vi "Main_Robot_Control2_j.vi"() -> ()   [LabVIEW 2014]
uses:
  <vilib>/Platform/TimedLoop/XDataNode/timing_clust.ctl
  <vilib>/Platform/TimedLoop/XDataNode/nitl_modes.ctl
  <vilib>/Platform/TimedLoop/XDataNode/wakeup.ctl
  <vilib>/Platform/TimedLoop/XDataNode/XDataNode.xnode
  <vilib>/Platform/TimedLoop/XDataNode/XDNodeRunTimeDep.lvlib
panel:
  in  "Subpanel Stop":bool
  out "Previous Iteration Finished Late?  2":bool
  out "Subpanel Running":bool
  out "Pot_D":dynamicdata(graph)
  out "IR_V":dynamicdata(graph)
  out "IR_D":dynamicdata(graph)
  out "Numeric":dbl
  out "Numeric 2":dbl
  out "Pot_V":dynamicdata(graph)
  out "stop 3":bool
  in  "stop 2":bool
  out "Boolean":bool
  in  "motor direction":bool
  in  "Set Start Posiotn of Head in Steps":dbl format="%#_13g"
  in  "Tab Control":T1(tab)
  out "Center IR":dbl(slide) scale=0.0..10.0
  out "Pot":dbl(slide) scale=0.0..10.0
  out "Gauge":dbl(knob) scale=0.0..10.0
  in  "Motor Direction":bool
  in  "Potentiometer":dbl(slide) scale=0.0..5.0
  out "Previous Iteration Finished Late?":bool
  # "E-STOP"
  # "See the block diagram for modification instructions."
  # "CCW"
  # "CCW"
  # "CW"
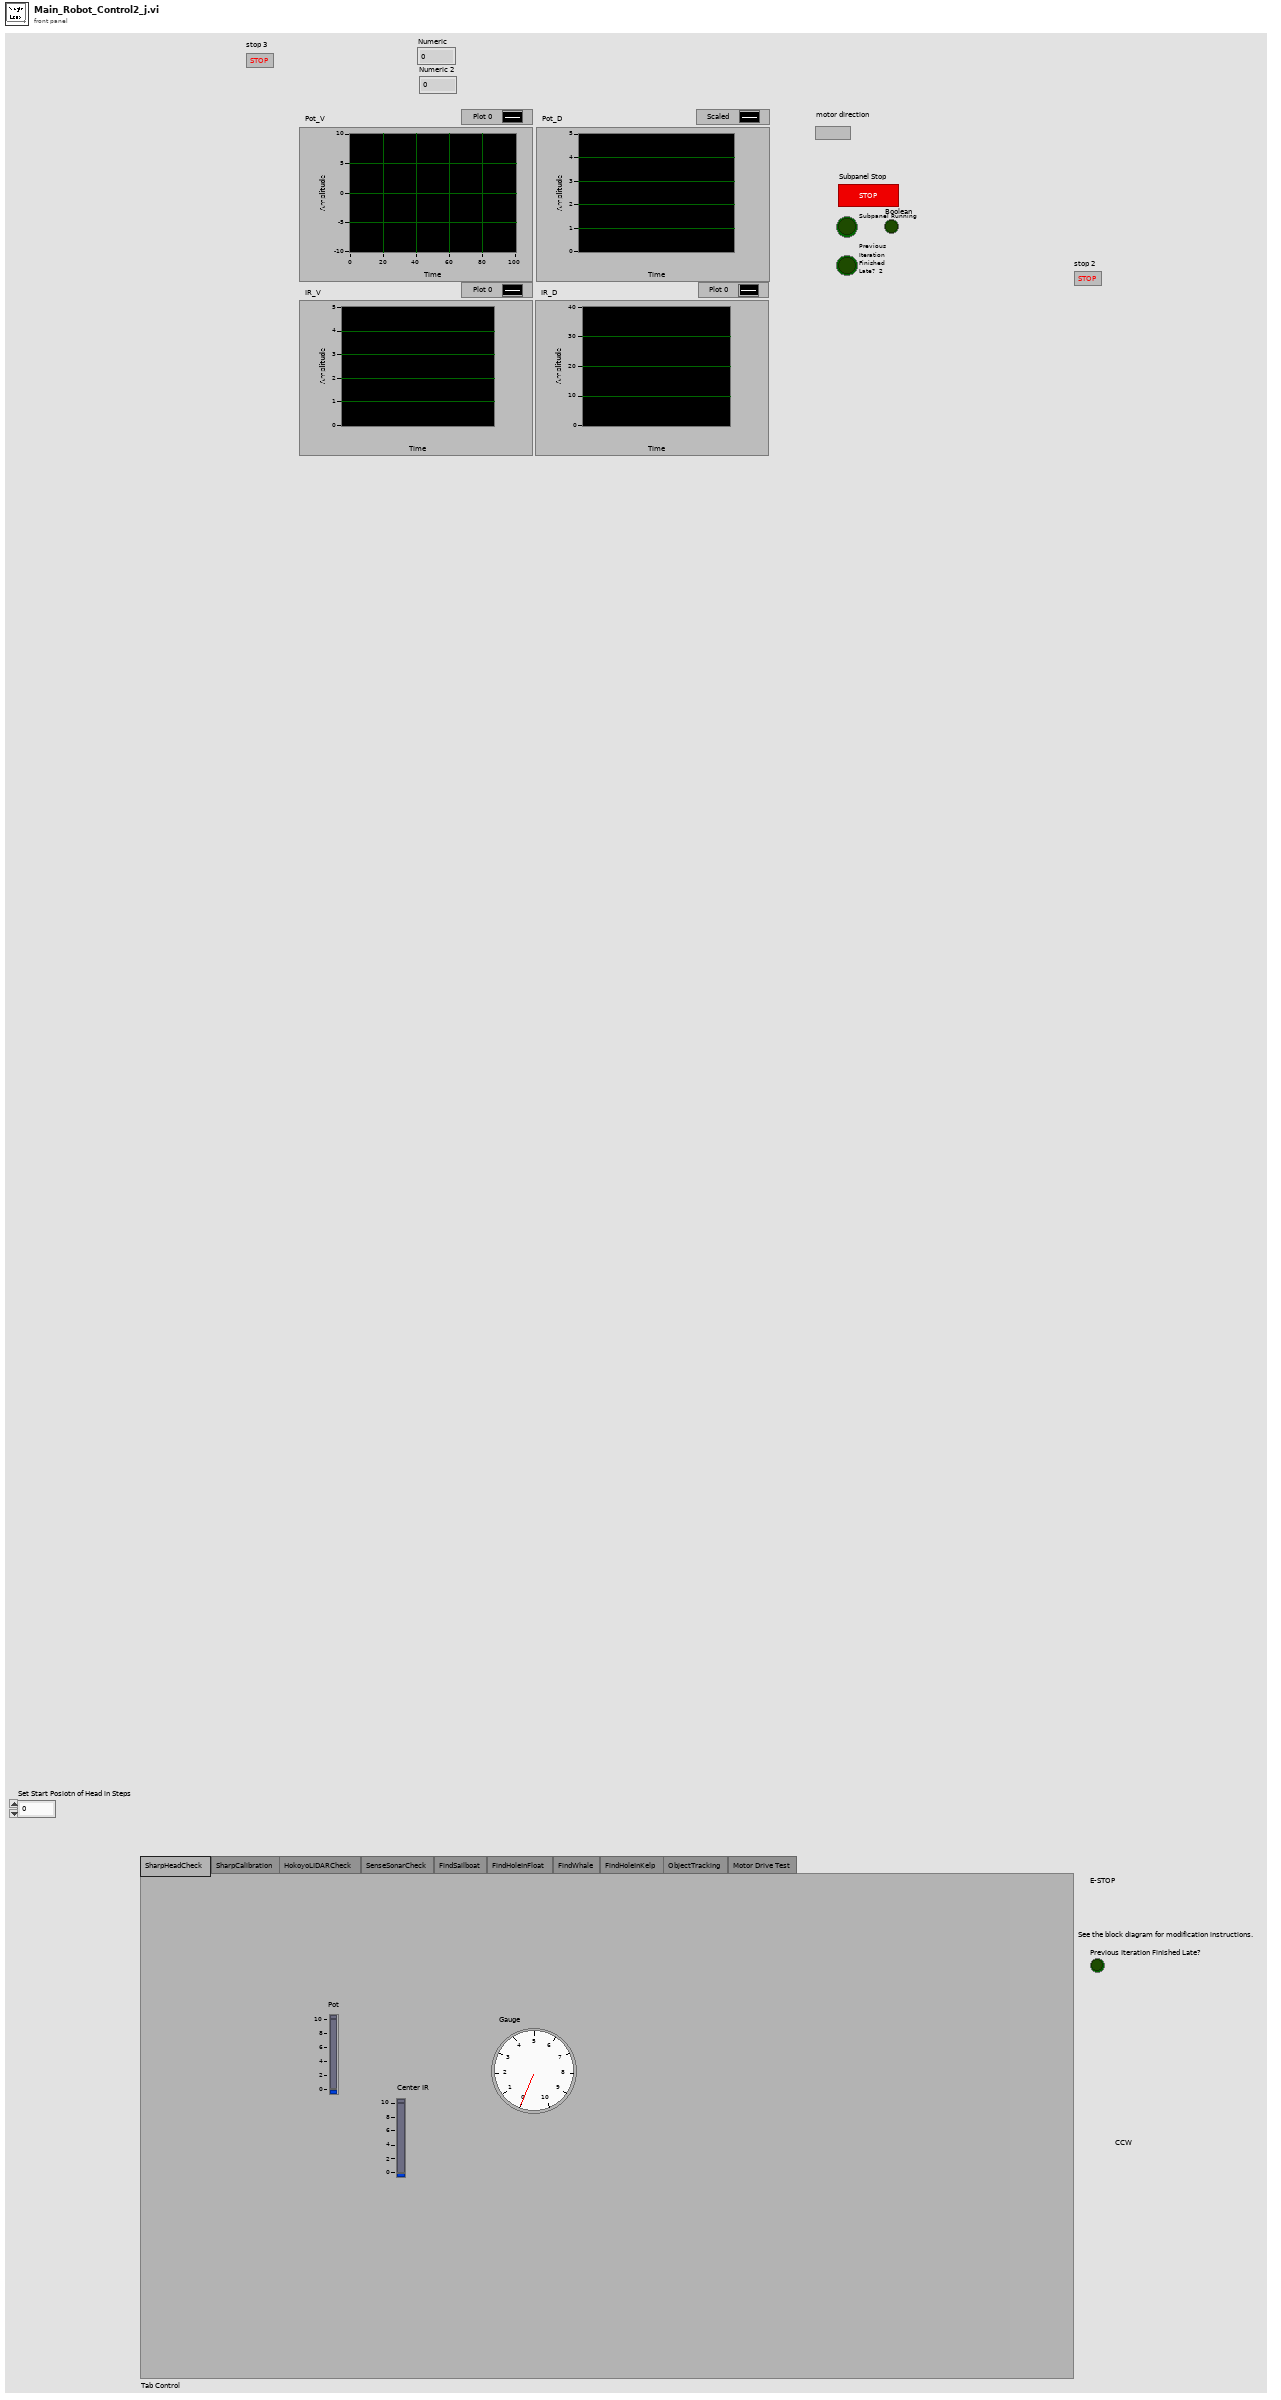
[diagram p1: front panel]
types:
  T1 = enum32{"SharpHeadCheck", "SharpCalibration", "HokoyoLIDARCheck", "SenseSonarCheck", "FindSailboat", "FindHoleInFloat", "FindWhale", "FindHoleInKelp", "ObjectTracking", "Motor Drive Test"}
  T2 = typedef "XDNodeRunTimeDep.lvlib/timing_clust.ctl" = cluster{"Expected End [f-1]":u64, "Actual End [f-1]":u64, "Finished Late? [f-1]":bool, "Expected End [i-1]":u64, "Actual End [i-1]":u64, "Finished Late? [i-1]":bool, "Expected Start [i]":u64, "Actual Start [i]":u64, "Expected Start [f]":u64, "Actual Start [f]":u64, "Source Name":string, "Structure Name":string, "Period":i64, "Deadline":i64, "Offset":i64, "Start":i64, "Priority":i32, "Timeout":i32, "Mode":T3, "Wakeup Reason":T4, "Error":errorcluster, "Source Type":string, "Secondary Source Type":string, "Global End Time":u64, "Global Start Time":u64, "Frame Duration":u64, "Iteration Duration":u64, "Assigned CPU":i32, "I/O Scan Engine Mode":u32}
  T3 = typedef "XDNodeRunTimeDep.lvlib/nitl_modes.ctl" = enum32{"No Change", "Process missed periods, maintain original phase", "Discard missed periods, maintain original phase", "Process missed periods, ignore original phase", "Discard missed periods, ignore original phase"}
  T4 = typedef "XDNodeRunTimeDep.lvlib/wakeup.ctl" = enum32{"Normal", "Aborted", "Asynchronous wakeup", "Timing source error", "Timed loop error", "Timeout"}
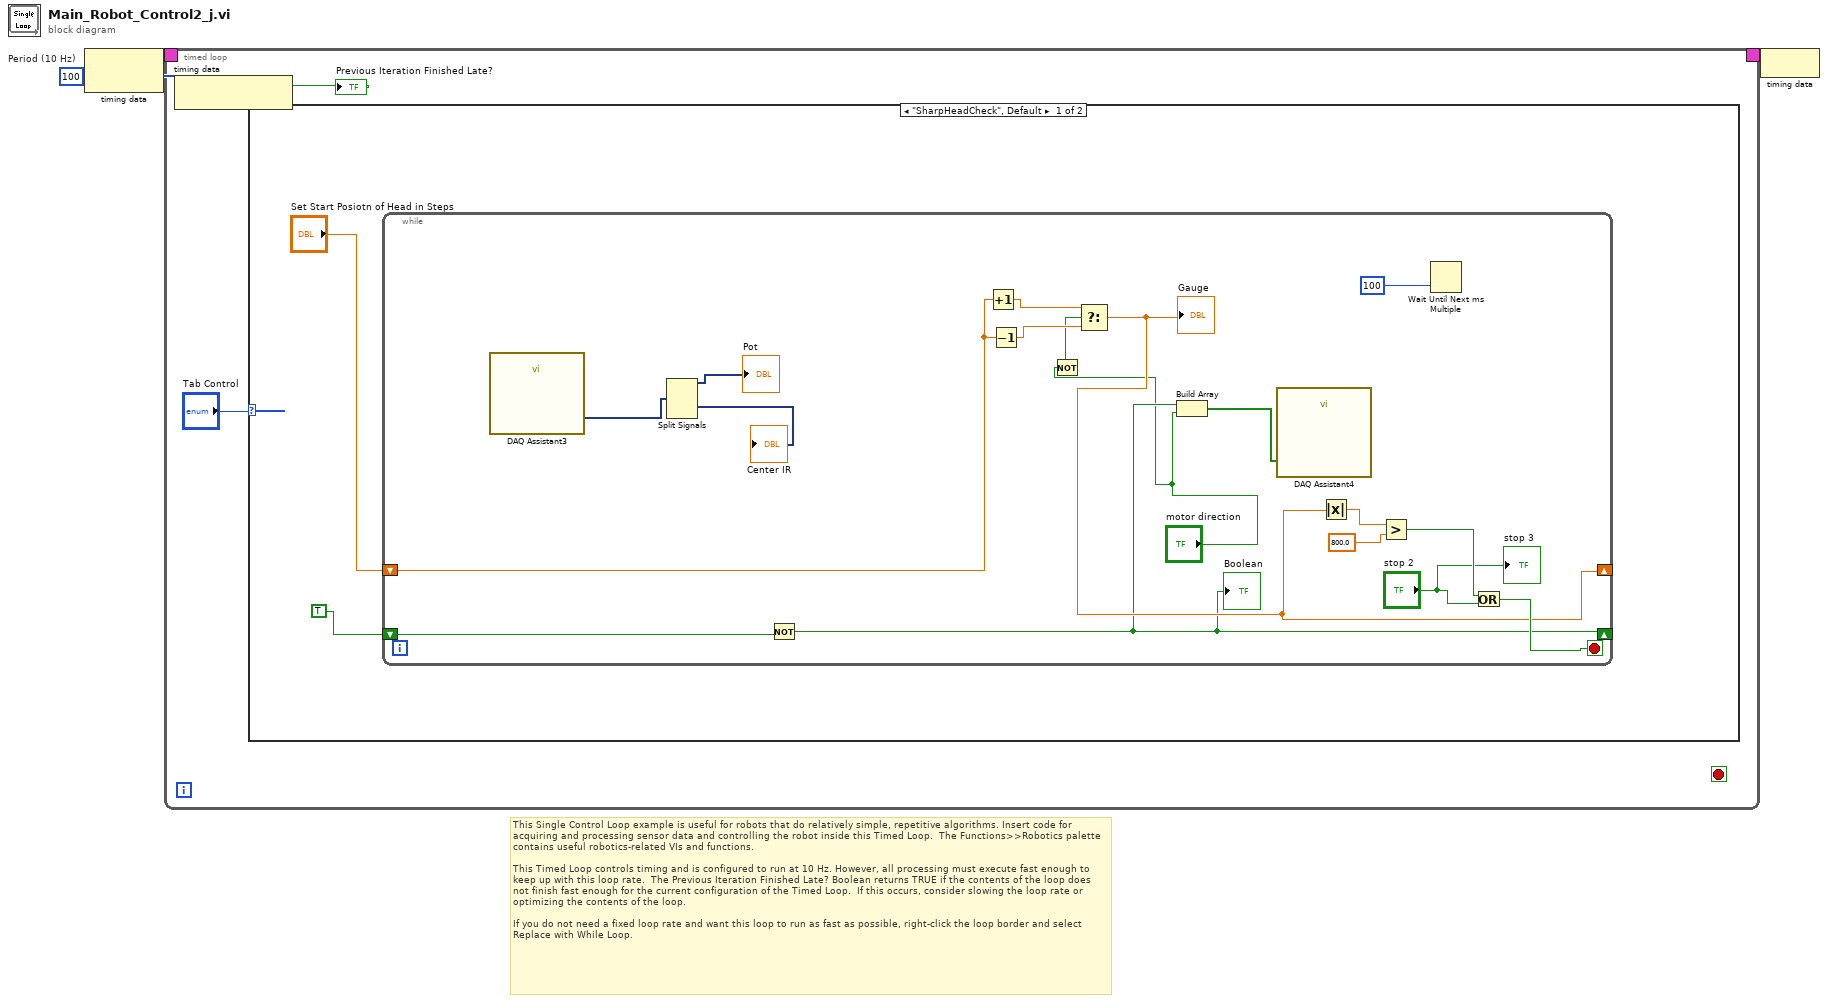
[diagram p0: block diagram]
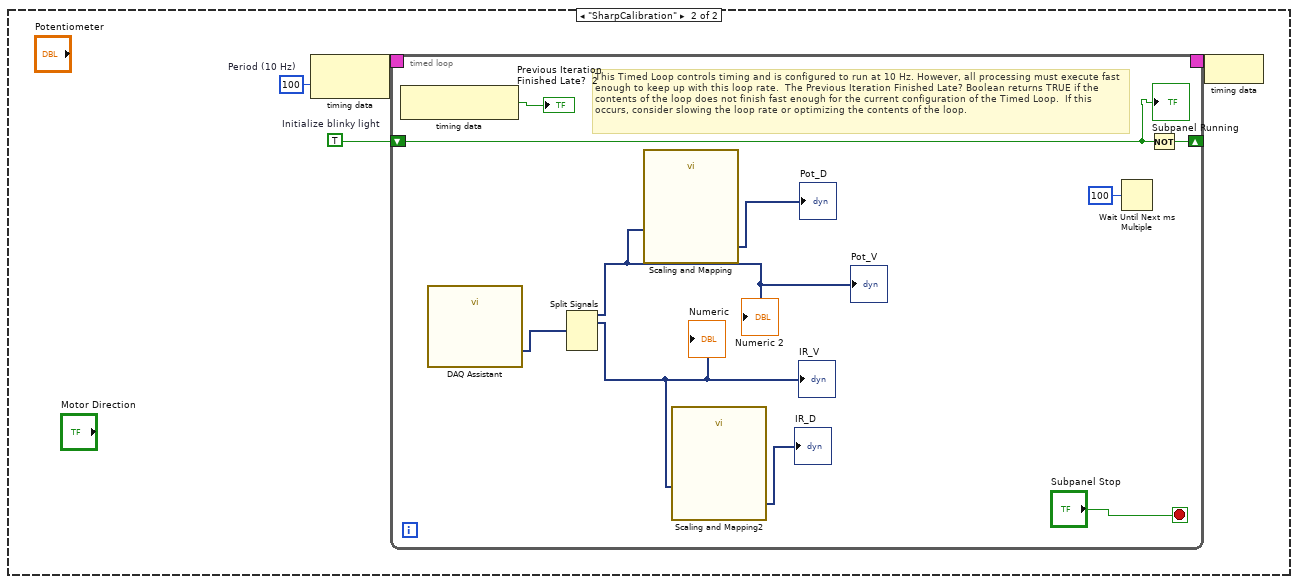
[diagram p2: hidden frame]
diagram:
  w1 = i64 100  # Period (10 Hz)
  # "This Single Control Loop example is useful for robots that do relatively simple, repetitive algorithms. Insert code for acquiring and processing sensor data and controlling the robot inside this Timed Loop.  The Functions>>Robotics palette contains useful robotics-related VIs and functions.\n\nThis Timed Loop controls timing and is configured to run at 10 Hz. However, all processing must execute fast enough to keep up with this loop rate.  The Previous Iteration Finished Late? Boolean returns TRUE if the contents of the loop does not finish fast enough for the current configuration of the Timed Loop.  If this occurs, consider slowing the loop rate or optimizing the contents of the loop.\n\nIf you do not need a fixed loop rate and want this loop to run as fast as possible, right-click the loop border and select Replace with While Loop."
  n1 = node-c288(w1) -> (w3:T2)
  n2 = timed-loop {
    timing: w3 -> [_]
    timing-out: [_] -> w2
    stop <- _ stop-if-true
    n3 = node-c288() -> (→"Previous Iteration Finished Late?":bool)  [unwired: 1 in]
    n4 = case shown="\"SharpHeadCheck\", Default" "Tab Control" {
      frame "SharpHeadCheck", Default {
        n5 = while {
          shift-right: [w13] -> _
          shift-left: TRUE -> [w18]
          shift-right: [w14] -> _
          shift-left: "Set Start Posiotn of Head in Steps" -> [w25]
          stop <- w22 stop-if-true
          n6 = call "DAQ Assistant3"() -> ("data"=w16:dynamicdata)  [unwired: 17 in, 2 out]
          n7 = Split Signals(w16) -> (→"Pot":dynamicdata, →"Center IR":dynamicdata)  [unwired: 5 in, 3 out]
          n8 = Not(x=w18) -> (.not. x?=w13:bool)
          "Boolean" <- w13
          n9 = Increment(x=w25) -> (x+1=w23:dbl)
          n10 = Decrement(x=w25) -> (x-1=w24:dbl)
          n11 = Not(x="motor direction") -> (.not. x?=w10:bool)
          n12 = Select(t=w23, s=w10, f=w24) -> (s? t:f=w14:dbl)
          "Gauge" <- w14
          n13 = Build Array(w13, "motor direction") -> (w15:bool[])
          n14 = call "DAQ Assistant4"("data"=w15) -> ()  [unwired: 17 in, 2 out]
          n15 = Absolute Value(x=w14) -> (abs(x)=w19:dbl)
          n16 = Greater?(x=w19, y=800.0) -> (0:w21:bool)
          n17 = Wait Until Next ms Multiple(millisecond multiple=u32 100 ("millisecond timer value")) -> ()  [unwired: 1 out]
          n18 = Or(x=w21, y="stop 2") -> (x .or. y?=w22:bool)
          "stop 3" <- "stop 2"
        }
      }
      frame "SharpCalibration" {
        w26 = TRUE  # Initialize blinky light
        w27 = i64 100  # Period (10 Hz)
        n19 = node-c288(w27) -> (w29:T2)
        n20 = timed-loop {
          timing: w29 -> [_]
          timing-out: [_] -> w28
          shift-right: [w39] -> _
          shift-left: w26 -> [w36]
          stop <- "Subpanel Stop" stop-if-true
          # "This Timed Loop controls timing and is configured to run at 10 Hz. However, all processing must execute fast enough to keep up with this loop rate.  The Previous Iteration Finished Late? Boolean returns TRUE if the contents of the loop does not finish fast enough for the current configuration of the Timed Loop.  If this occurs, consider slowing the loop rate or optimizing the contents of the loop."
          n21 = node-c288() -> (→"Previous Iteration Finished Late?  2":bool)  [unwired: 1 in]
          n22 = call "DAQ Assistant"() -> ("data"=w32:dynamicdata)  [unwired: 17 in, 2 out]
          n23 = Split Signals(w32) -> (w30:dynamicdata, w31:dynamicdata)  [unwired: 5 in, 3 out]
          "IR_V" <- w31
          "Numeric" <- w31
          "Numeric 2" <- w30
          "Pot_V" <- w30
          n24 = call "Scaling and Mapping"("Signals"=w30) -> ("Scaled Signals"=→"Pot_D":dynamicdata)  [unwired: 9 in, 1 out]
          n25 = call "Scaling and Mapping2"("Signals"=w31) -> ("Scaled Signals"=→"IR_D":dynamicdata)  [unwired: 9 in, 1 out]
          n26 = Wait Until Next ms Multiple(millisecond multiple=u32 100) -> ()  [unwired: 1 out]
          n27 = Not(x=w36) -> (.not. x?=w39:bool)
          "Subpanel Running" <- w36
        }
        n28 = node-c288(w28) -> ()
      }
    }
  }
  n29 = node-c288(w2) -> ()
